vi "Set Power.vi"(8 "error in (no error)":errorcluster, 11 "Harmonics in":refnum<class "Harmonics.lvclass">) -> (0 "error out":errorcluster, 1 "Parameter":cluster{"Name":string, "Value":string}, 2 "Last Power?":bool, 3 "Harmonics out":refnum<class "Harmonics.lvclass">)   [LabVIEW 2020, in "Harmonics.lvclass"]
uses:
  Harmonics.lvclass
  Harmonics.lvclass/Harmonics.ctl
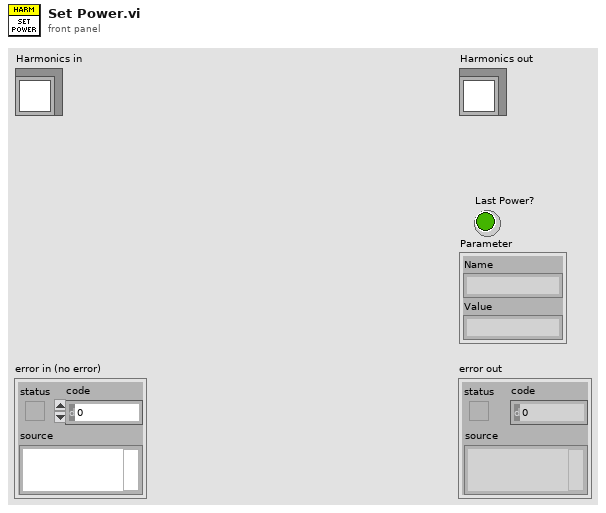
[diagram p1: front panel]
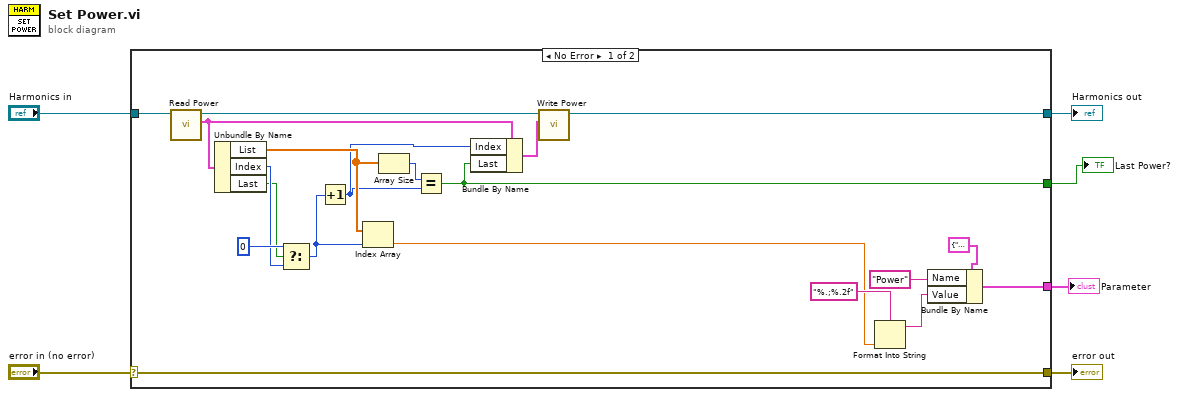
[diagram p0: block diagram]
diagram:
  n1 = case shown="No Error" "error in (no error)" {
    selector: "error in (no error)" -> [w8 w28]
    tunnel: [w8 w28] -> w5
    tunnel: [w7 w27] -> w3
    tunnel: "Harmonics in" -> [w9 w27]
    tunnel: [w16 _] -> w2
    tunnel: [w10 _] -> w1
    frame No Error {
      n2 = call "Read Power.vi"("Harmonics in"=w9) -> ("Power"=w25:cluster{"List":dbl[], "Index":i32, "Last":bool}, "Harmonics out"=w26:refnum<class "Harmonics.lvclass">)  [unwired: 9 in]
      n3 = Unbundle By Name(w25) -> ("List"=w20:dbl[], "Index"=w23:i32, "Last"=w21:bool)
      n4 = Select(t=0, s=w21, f=w23) -> (s? t:f=w18:i32)
      n5 = Increment(x=w18) -> (x+1=w17:i32)
      n6 = Index Array(array=w20, index=w18) -> (element=w11:dbl)
      n7 = Array Size(array=w20) -> (size(s)=w19:i32)
      n8 = Equal?(x=w19, y=w17) -> (x = y?=w16:bool)
      n9 = Bundle By Name(cluster=w25, "Index"=w17, "Last"=w16) -> (w22:cluster{"List":dbl[], "Index":i32, "Last":bool})
      n10 = call "Write Power.vi"("Power"=w22, "Harmonics in"=w26) -> ("Harmonics out"=w7:refnum<class "Harmonics.lvclass">)  [unwired: 9 in]
      n11 = Format Into String(format string="%.;%.2f", w11) -> (resulting string=w12:string)  [unwired: 2 in, 1 out]
      n12 = Bundle By Name(cluster=cluster{"Name":string, "Value":string} {"Name"="", "Value"=""} ("Change"), "Name"="Power", "Value"=w12) -> (w10:cluster{"Name":string, "Value":string})
    }
    frame Error {
    }
  }
  "error out" <- w5
  "Harmonics out" <- w3
  "Last Power?" <- w2
  "Parameter" <- w1
